vi "Teleop.vi"(10 "Match Info":T2={"Autonomous Elapsed Seconds"=0.0, "TeleOp Elapsed Seconds"=0.0, "Disabled Elapsed Seconds"=0.0, "Visited Autonomous"=FALSE, "Visited TeleOp"=FALSE, "Visited Disabled"=FALSE, "Autonomous Settings"={"Autonomous Style"=enum."Independent", "VI Refnum"=refnum}}, 11 "Call Context":T3) -> ()   [LabVIEW 2018]
doc: "This VI is called for each TeleOp packet received from the DS where the robot is not disabled. It is often used to read from the joysticks and update I/O or to update setpoints for timed control loops. It should complete and return within 20 milliseconds or it may miss DS packets."
uses:
  <vilib>/Rock Robotics/WPI/DriverStation/WPI_DriverStationDerivedRobotMode.ctl
  <vilib>/Rock Robotics/WPI/DriverStation/WPI_DriverStationMatch Info.ctl
  <vilib>/Rock Robotics/WPI/ThirdParty/Phoenix-LabVIEW/Motor Controller/Controls/CTRE_Phoenix_MotorControl_ControlMode.ctl
  <vilib>/Rock Robotics/WPI/Solenoid/WPI_SolenoidValue.ctl
  <vilib>/Rock Robotics/WPI/Utilities/WPI_GetSetVariantRefNum.vi
  <vilib>/Rock Robotics/WPI/ThirdParty/Phoenix-LabVIEW/Motor Controller/Get/CTRE_Phoenix_MotorController_GetSelectedSensorData.vi
  <vilib>/Rock Robotics/WPI/Solenoid/WPI_SolenoidSetEnum.vi
  <vilib>/Rock Robotics/Network Tables/NT Read Number.vi
panel:
  in  "FollowerLeft":dbl(slide) scale=-1.0..1.0
  in  "spark6":dbl(slide) scale=-1.0..1.0
  in  "Send LED Byte":bool
  in  "LED Byte":string
  out "Num Bytes Written":u32
  out "Operator Axis 4":dbl(slide) scale=-1.0..1.0
  out "Operator Buttons":bool[](array[boolean])
  out "Operator Axis 3":dbl(slide) scale=-1.0..1.0
  out "Operator Axis 2":dbl(slide) scale=-1.0..1.0
  out "Operator Axis 1":dbl(slide) scale=-1.0..1.0
  out "Image Out":T1(plugin-control)
  out "spark6encoder":dbl
  out "spark5encoder":dbl
  out "MasterLeft":dbl
  out "FollowerLeft":dbl
  out "MasterRight":dbl
  out "FollowerRight":dbl
  out "Keyboard Data":dbl
  out "HorseRight":i32
  out "ElevatorLeft":i32
  out "IntakeWrist":i32
  in  "Butterfly Drive Control":bool
  in  "Individual\nControl":bool
  in  "Test Run":bool
  in  "CargoKicker":bool
  in  "HorseDriveHatch":bool
  in  "Hatch":bool
  in  "Butterfly":bool
  in  "HorseLift":dbl(slide) scale=-1.0..1.0
  in  "IntakeWheels":dbl(slide) scale=-1.0..1.0
  in  "IntakeWrist":dbl(slide) scale=-1.0..1.0
  in  "ElevatorRight":dbl(slide) scale=-1.0..1.0
  in  "ElevatorLeft":dbl(slide) scale=-1.0..1.0
  in  "OuterStageDrive":dbl(slide) scale=-1.0..1.0
  in  "spark5":dbl(slide) scale=-1.0..1.0
  in  "MasterLeft":dbl(slide) scale=-1.0..1.0
  in  "MasterRight":dbl(slide) scale=-1.0..1.0
  in  "FollowerRight":dbl(slide) scale=-1.0..1.0
  # "TO DO LIST:\nUpdate all Talons and Victors\nto most recent firmware version\n4.17 for both controllers, firmware\nis located under 2019 firmware folder.\n\nID all motor controllers. Current code\nassumes the following ID's:\n0/1=LeftDrive\n2/3=RightDrive\n4=ButterflyLeft\n5=ButterflyRight\n6=OuterStage\n7=ElevatorLeft\n8=ElevatorRight\n9=IntakeWrist\n10=IntakeWheelse\n11=HorseDriveLeft\n12=HorseDriveRight\n\nVerify solenoid and PCM ID's, current\ncode assumes the following ID's:\n15=PCM\nSolenoid 0/1=Butterfly (dbl)\nSolenoid 2/3=Shift (dbl)\nSolenoid 4=Hatch (sngle)\nSolenoid 5=HorseDriveHatch (sngle)\nSolenoid 6=CargoKicker (sngle)"
  # "ADDITIONAL INFORMATION:\nCurrent code assumes all Talons for \nnon-drive-train motors. If some are\nVictors you only need to replace the open\nTalon VI's in BEGIN, all other VI's, such as\nset value, get value, refnum set/get, etc. \nare the same between Victor's or Talons.\n\nCurrent code has inverted the following:\nspark1\nspark2\nspark5\nElevatorRight\nHorseDriveRight\n\nThe main robot code uses the same\nbegin and finish code as the test project,\nTele-op however looks very different \nand uses keyboard based operator\nstation, if ready switch the operator station\nto a standard joystick copying off of the \nexisting joystick code. In addition, in the \nteleop there are two disabled VI's, the lower\none moved the elevator to a set encoder \nvalue and the other is a line following\ntest program. Both are completly untested\nfirst drafts use with caution. They are the \nlowest priorty to test."
  # "Controls main drive REV motors. 0 means\nno motor power, -1 means full reverse,1 means full \nforward. Spark 0-1 should ber ight drive, Spark 2-3 \nshould be left drive, Spark 4-5 should be butterfly \ndrive, with 4 being the left one.If individual control \nis TRUE, each slider controls that motor. If individual \ncontrol is FALSE, the slider becomes an indicator that \ndisplays percent output each motor is getting from \nthe joystick."
  # "Boolean control for\neach solenoid:\nTRUE: solenoid runs forward\nif doubleacting, or on if single\nacting. Should extend the piston.\nFALSE: Solenoid runs reverse if \ndoubleacting, or off if single\nacting, should withdraw the piston."
  # "Displays all axis from the operator station"
  # "Displays operator\nstation button\nvalues."
  # "Displays image fed into teleop from vision processing.VI"
  # "All encoder data from each\nREV Motor internal encoder"
  # "Controls LED signals"
  # "Sliders control talon motors, 0 means\nno motor power, -1 means full reverse,\n1 means full forward. \nIf Individual control is TRUE, this controls\neach specific motor, ignoring the other\nCAUTION,\nthis can damage gearboxes by running motors\nagainst each other\nIf Individual motor if FALSE, left (such as ElevatorLeft)\nmotor controls instead follow the right input."
  # "Test Run:\nFALSE: all functionality is disabled.\nTRUE: Allows robot control\n\nIndividiual Control\nFALSE: Controls elevator and horse\ndrive as one entity using the right\ninput, also drives the robot using\njoystick information.\nTRUE: Controls each motor directly\nand independitly from the others, CAUTION,\nthis can damage gearboxes by running motors\nagainst each other.\n\nButterfly Drive Control (Only has effect if\nIndividual control is FALSE).\nTRUE: Joystick control powers butterfly drive\nFALSE: Joystick control powers standard drive."
  # "All mag encoder data recieved from the robot, alongside\ncurrent keyboard data detected from dashboard."
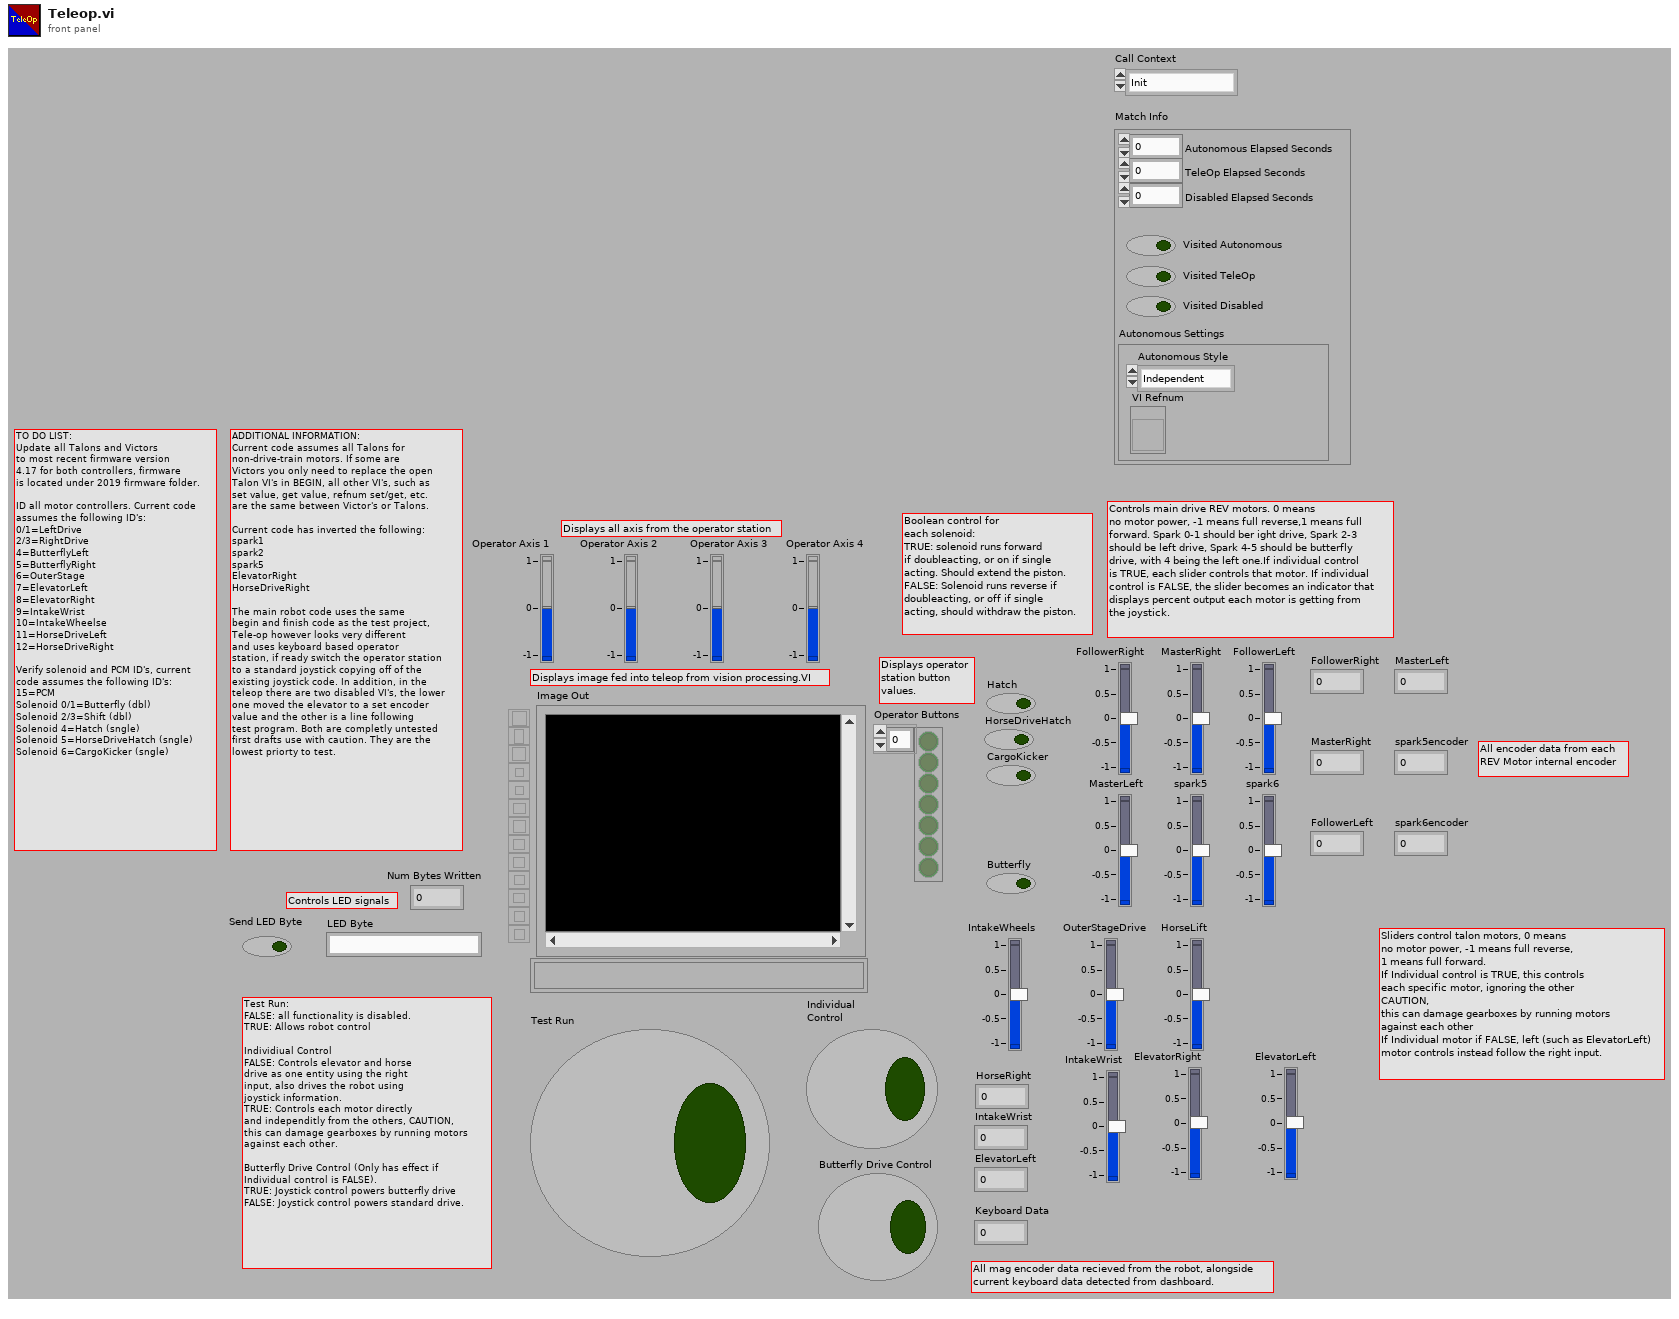
[diagram p1: front panel]
types:
  T1 = typedef "IMAQ Image.ctl" = refnum<image>
  T2 = typedef "WPI_DriverStationMatch Info.ctl" = cluster{"Autonomous Elapsed Seconds":dbl, "TeleOp Elapsed Seconds":dbl, "Disabled Elapsed Seconds":dbl, "Visited Autonomous":bool, "Visited TeleOp":bool, "Visited Disabled":bool, "Autonomous Settings":cluster{"Autonomous Style":enum16{"Iterative", "Independent"}, "VI Refnum":refnum<vi>}}
  T3 = typedef "WPI_DriverStationDerivedRobotMode.ctl" = enum16{"Init", "Execute", "Stop"}
  T4 = typedef "WPI_SerialPortRef.ctl" = cluster{"DevStatus":errorcluster, "Serial Port Name":refnum<visa-resource-name>}
  T5 = typedef "WPI_SolenoidValue.ctl" = enum16{"Off", "On", "Forward", "Reverse"}
  T6 = typedef "CTRE_Phoenix_MotorControl_ControlMode.ctl" = u16
  T7 = typedef "WPI_MotorControlDeviceRef.ctl" = cluster{"DeviceStatus":errorcluster, "Type":T8, "PWM":cluster{"PWM Channel":T9, "DeadBand":T10}, "CAN":cluster{"Device Number":u8, "SetOutput VI Ref":variant, "GetOutput VI Ref":variant, "Enable VI Ref":variant, "Disable VI Ref":variant, "Data":variant}, "Invert":bool, "DIO PWM":cluster{"PWM \"Enable\" Channel":T9, "DIOChannel":T11, "PWM Rate":dbl}}
  T8 = typedef "WPI_MotorControlType.ctl" = enum16{"PWM", "CAN", "DIO PWM"}
  T9 = typedef "FPGA_DIOPWMChannel.ctl" = enum8{"PWM 0", "PWM 1", "PWM 2", "PWM 3", "PWM 4", "PWM 5", "PWM 6", "PWM 7", "PWM 8", "PWM 9", "PWM MXP 0", "PWM MXP 1", "PWM MXP 2", "PWM MXP 3", "PWM MXP 4", "PWM MXP 5", "PWM MXP 6", "PWM MXP 7", "PWM MXP 8", "PWM MXP 9", "Invalid"}
  T10 = typedef "WPI_PWMDeadband.ctl" = cluster{"Name":string, "maxPositivePwm":i32, "minPositivePwm":i32, "centerPwm":i32, "maxNegativePwm":i32, "minNegativePwm":i32, "angularRange":u16}
  T11 = typedef "FPGA_DIOChannel.ctl" = enum8{"DIO 0", "DIO 1", "DIO 2", "DIO 3", "DIO 4", "DIO 5", "DIO 6", "DIO 7", "DIO 8", "DIO 9", "DIO MXP 0", "DIO MXP 1", "DIO MXP 2", "DIO MXP 3", "DIO MXP 4", "DIO MXP 5", "DIO MXP 6", "DIO MXP 7", "DIO MXP 8", "DIO MXP 9", "DIO MXP 10", "DIO MXP 11", "DIO MXP 12", "DIO MXP 13", "DIO MXP 14", "DIO MXP 15", "SPI Port CS1", "SPI Port CS2", "SPI Port CS3", "SPI Port MISO", "SPI Port MOSI", "Invalid"}
  T12 = typedef "WPI_JoystickDevRef.ctl" = cluster{"Device":T13}
  T13 = typedef "WPI_JoystickDeviceEnum.ctl" = enum16{"USB 0", "USB 1", "USB 2", "USB 3", "USB 4", "USB 5"}
  T14 = typedef "WPI_CameraDevRef.ctl" = cluster{"Camera Address":string, "CameraStatus":errorcluster}
  T15 = typedef "WPI_SolenoidDevRef.ctl" = cluster{"DevStatus":errorcluster, "Pneumatics Control Module":u8, "Forward Solenoid Channel":T16, "Reverse Solenoid Channel":T16}
  T16 = typedef "WPI_SolenoidChannel.ctl" = enum8{"Solenoid 0", "Solenoid 1", "Solenoid 2", "Solenoid 3", "Solenoid 4", "Solenoid 5", "Solenoid 6", "Solenoid 7", "Invalid"}
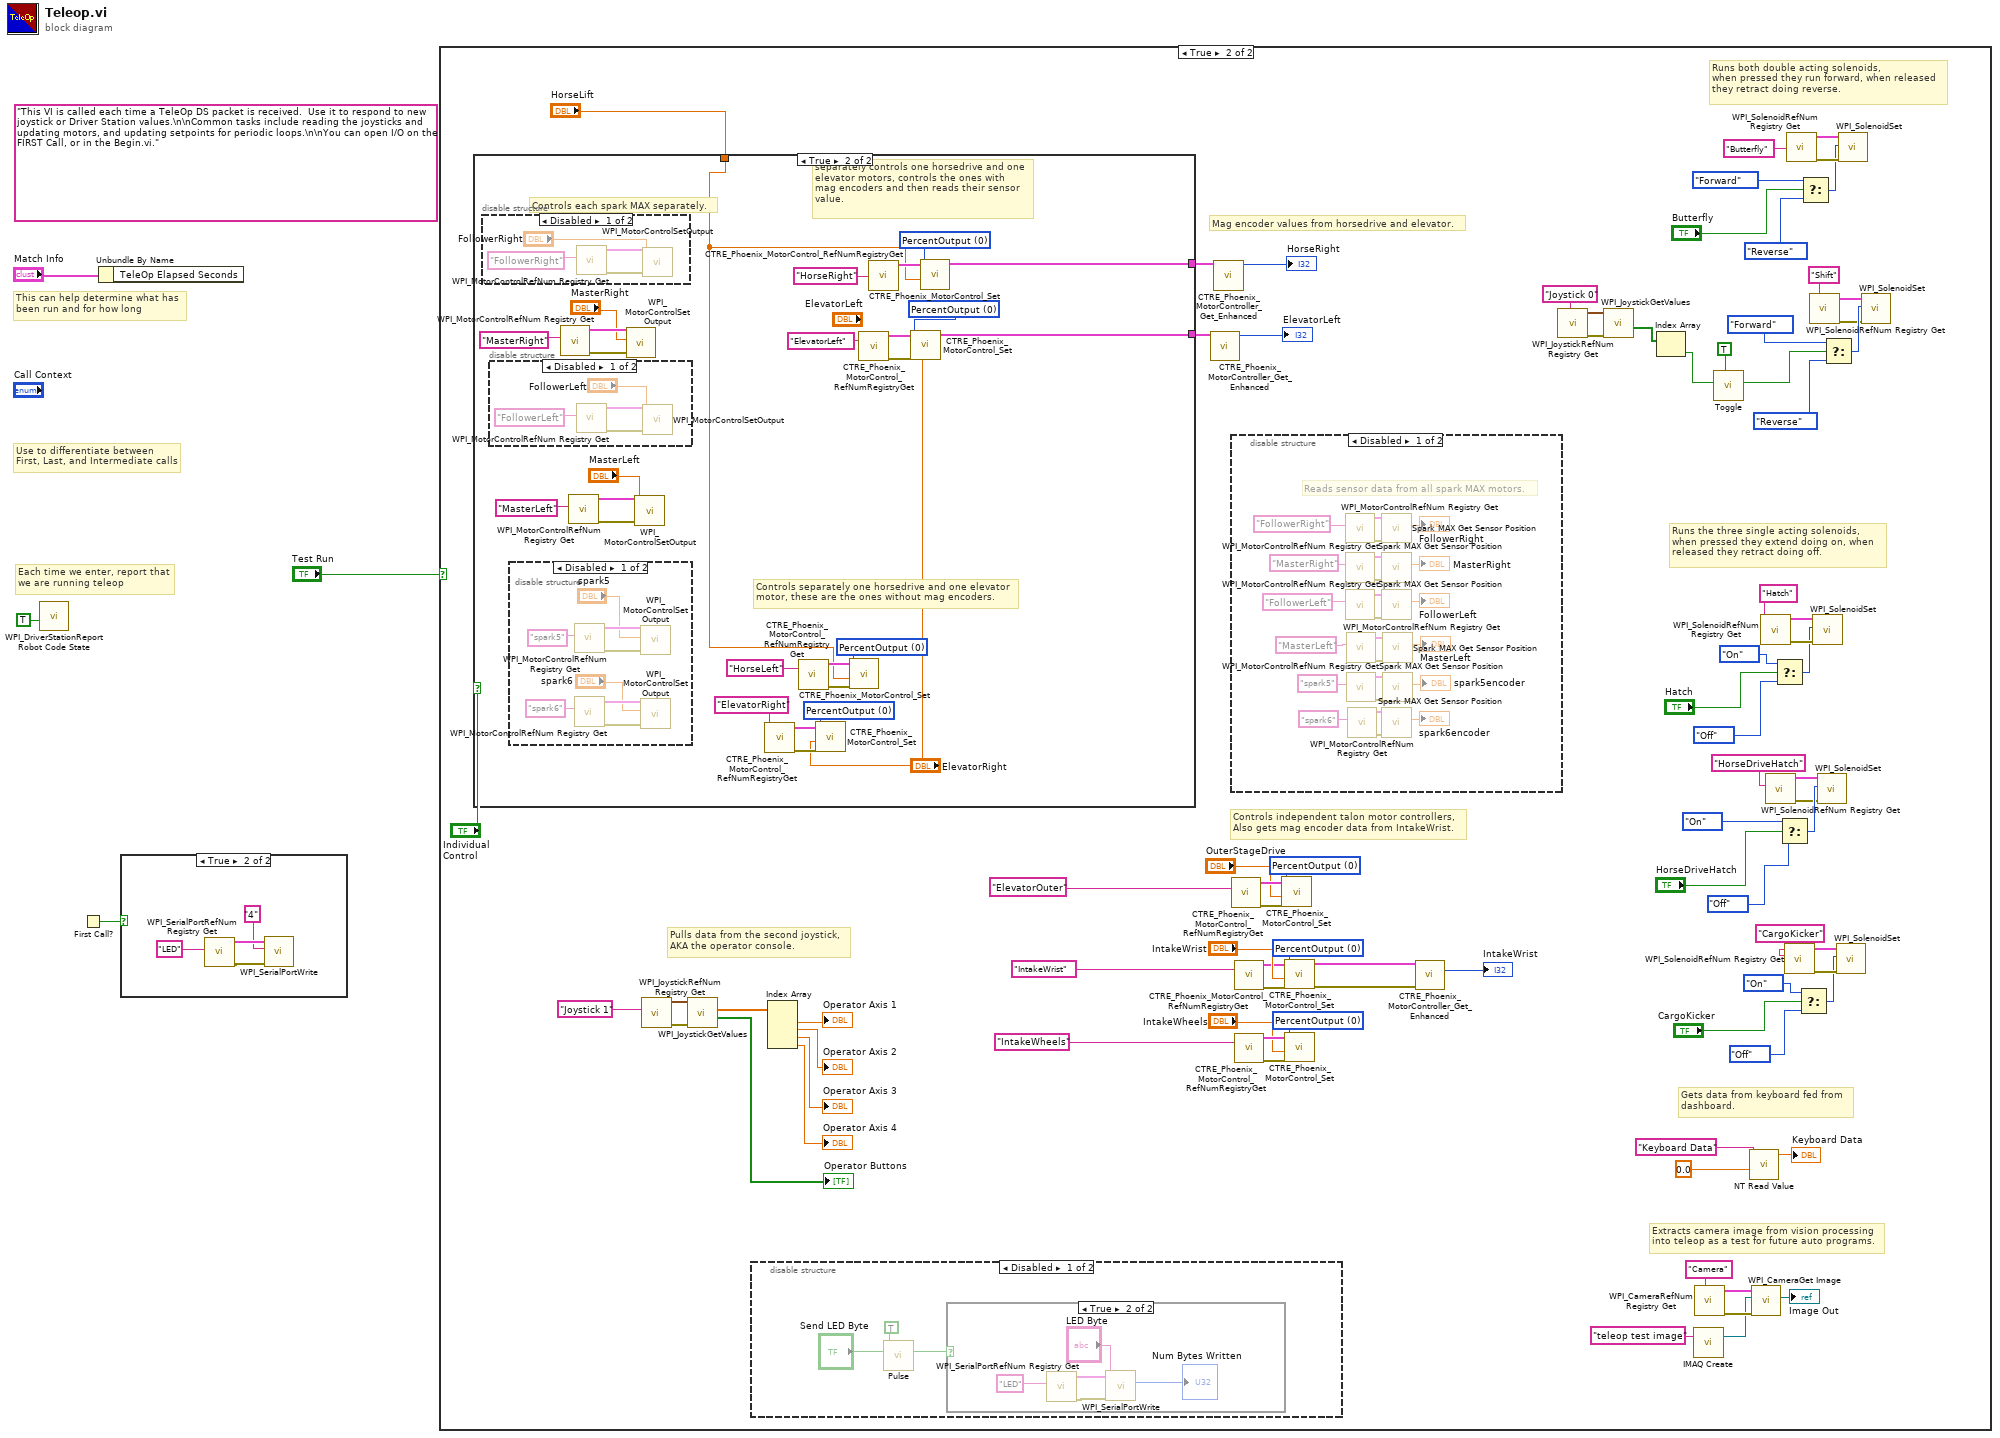
[diagram p0: block diagram]
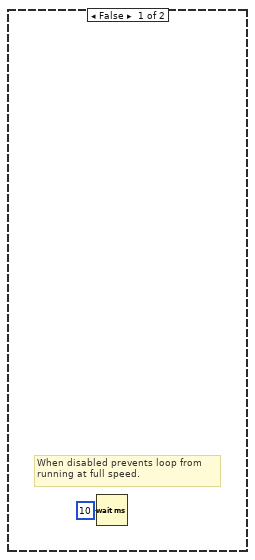
[diagram p3: hidden frame]
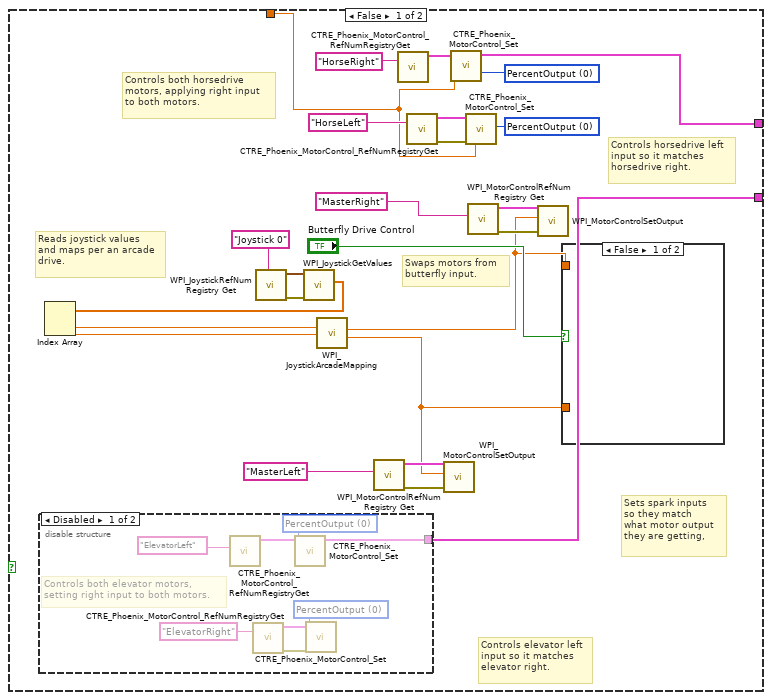
[diagram p7: hidden frame]
diagram:
  (unwired) "This VI is called each time a TeleOp DS packet is received.  Use it to respond to new joystick or Driver Station values.\n\nCommon tasks include reading the joysticks and updating motors, and updating setpoints for periodic loops.\n\nYou can open I/O on the FIRST Call, or in the Begin.vi."
  # "Each time we enter, report that\nwe are running teleop"
  # "Use to differentiate between\nFirst, Last, and Intermediate calls"
  # "This can help determine what has\nbeen run and for how long"
  n1 = call <vilib>:"WPI_DriverStationReport Robot Code State.vi"("TeleOp"=TRUE ("Autonomous")) -> ()  [unwired: 10 in, 1 out]
  n2 = First Call?() -> (First Call?: T/F=w1:bool)
  n3 = Unbundle By Name("Match Info") -> ()  [unwired: 1 out]
  n4 = case shown="True" w1 {
    frame False {
    }
    frame True {
      n5 = call <vilib>:"WPI_SerialPortRefNum Registry Get.vi"("refnum name"="LED") -> ("error out"=w5:errorcluster, "SerialPortRef"=w7:T4)  [unwired: 9 in]
      n6 = call <vilib>:"WPI_SerialPortWrite.vi"("error in (no error)"=w5, "Buffer"="4", "SerialPortRef"=w7) -> ()  [unwired: 6 in, 3 out]
    }
  }
  n7 = case shown="True" "Test Run" {
    frame False {
      # "When disabled prevents loop from\nrunning at full speed."
      n8 = Wait (ms)(milliseconds to wait=u32 10) -> ()  [unwired: 1 out]
    }
    frame True {
      w67 = T6 0 items=["PercentOutput"=0, "Position"=1, "Velocity"=2, "Current"=3, "Follower"=5, "MotionProfile"=6, "MotionMagic"=7, "MotionProfileArc"=10, "Disabled"=15] ("Control Mode")
      w72 = T6 0 items=["PercentOutput"=0, "Position"=1, "Velocity"=2, "Current"=3, "Follower"=5, "MotionProfile"=6, "MotionMagic"=7, "MotionProfileArc"=10, "Disabled"=15] ("Control Mode")
      w77 = T6 0 items=["PercentOutput"=0, "Position"=1, "Velocity"=2, "Current"=3, "Follower"=5, "MotionProfile"=6, "MotionMagic"=7, "MotionProfileArc"=10, "Disabled"=15] ("Control Mode")
      # "Mag encoder values from horsedrive and elevator."
      # "Extracts camera image from vision processing\ninto teleop as a test for future auto programs."
      # "Gets data from keyboard fed from\ndashboard."
      # "Runs both double acting solenoids,\nwhen pressed they run forward, when released\nthey retract doing reverse."
      # "Controls independent talon motor controllers,\nAlso gets mag encoder data from IntakeWrist."
      # "Pulls data from the second joystick,\nAKA the operator console."
      # "Runs the three single acting solenoids,\nwhen pressed they extend doing on, when\nreleased they retract doing off."
      n9 = case shown="True" "Individual\nControl" {
        tunnel: "HorseLift" -> [w127 w167]
        tunnel: [w131 w184] -> w90
        tunnel: [w132 w183] -> w89
        frame False {
          w134 = T6 0 items=["PercentOutput"=0, "Position"=1, "Velocity"=2, "Current"=3, "Follower"=5, "MotionProfile"=6, "MotionMagic"=7, "MotionProfileArc"=10, "Disabled"=15] ("Control Mode")
          w138 = T6 0 items=["PercentOutput"=0, "Position"=1, "Velocity"=2, "Current"=3, "Follower"=5, "MotionProfile"=6, "MotionMagic"=7, "MotionProfileArc"=10, "Disabled"=15] ("Control Mode")
          # "Sets spark inputs\nso they match\nwhat motor output\nthey are getting,"
          # "Controls horsedrive left\ninput so it matches \nhorsedrive right."
          # "Controls elevator left\ninput so it matches \nelevator right."
          # "Swaps motors from\nbutterfly input."
          # "Reads joystick values\nand maps per an arcade\ndrive."
          # "Controls both horsedrive\nmotors, applying right input\nto both motors."
          n10 = disable-structure shown="Disabled" {
            disable-tunnel: [w150 _] -> w131
            frame Disabled {
              w154 = T6 0 items=["PercentOutput"=0, "Position"=1, "Velocity"=2, "Current"=3, "Follower"=5, "MotionProfile"=6, "MotionMagic"=7, "MotionProfileArc"=10, "Disabled"=15] ("Control Mode")
              w157 = T6 0 items=["PercentOutput"=0, "Position"=1, "Velocity"=2, "Current"=3, "Follower"=5, "MotionProfile"=6, "MotionMagic"=7, "MotionProfileArc"=10, "Disabled"=15] ("Control Mode")
              # "Controls both elevator motors,\nsetting right input to both motors."
              n11 = call <vilib>:"CTRE_Phoenix_MotorControl_RefNumRegistryGet.vi"("refnum name"="ElevatorLeft") -> ("PhoenixMotorControlDevRef"=w151:T7)  [unwired: 9 in, 1 out]
              n12 = call <vilib>:"CTRE_Phoenix_MotorControl_RefNumRegistryGet.vi"("refnum name"="ElevatorRight") -> ("error out"=w156:errorcluster, "PhoenixMotorControlDevRef"=w155:T7)  [unwired: 9 in]
              n13 = call <vilib>:"CTRE_Phoenix_MotorControl_Set.vi"("Control Mode"=w157, "PhoenixMotorControlDevRef"=w151) -> ("PhoenixMotorControlDevRef"=w150:T7)  [unwired: 8 in, 1 out]
              n14 = call <vilib>:"CTRE_Phoenix_MotorControl_Set.vi"("error in (no error)"=w156, "Control Mode"=w154, "PhoenixMotorControlDevRef"=w155) -> ()  [unwired: 7 in, 2 out]
            }
            frame Enabled {
            }
          }
          n15 = call <vilib>:"WPI_JoystickRefNum Registry Get.vi"("refnum name"="Joystick 0") -> ("error out"=w145:errorcluster, "JoystickDevRef"=w144:T12)  [unwired: 9 in]
          n16 = call <vilib>:"WPI_JoystickGetValues.vi"("error in (no error)"=w145, "JoystickDevRef"=w144) -> ("Axes"=w142:dbl[])  [unwired: 5 in, 4 out]
          n17 = Index Array(array=w142) -> (element #1=w141:dbl, element #2=w140:dbl)  [unwired: 2 in]
          n18 = call <vilib>:"WPI_JoystickArcadeMapping.vi"("Y axis value"=w140, "X axis value"=w141) -> ("Right Motor Value"=w128:dbl, "Left Motor Value"=w129:dbl)  [unwired: 8 in]
          n19 = call <vilib>:"WPI_MotorControlRefNum Registry Get.vi"("refnum name"="MasterLeft") -> ("error out"=w149:errorcluster, "MotorControlDevRef"=w148:T7)  [unwired: 9 in]
          n20 = call <vilib>:"CTRE_Phoenix_MotorControl_RefNumRegistryGet.vi"("refnum name"="HorseRight") -> ("PhoenixMotorControlDevRef"=w135:T7)  [unwired: 9 in, 1 out]
          n21 = call <vilib>:"CTRE_Phoenix_MotorControl_RefNumRegistryGet.vi"("refnum name"="HorseLeft") -> ("error out"=w136:errorcluster, "PhoenixMotorControlDevRef"=w137:T7)  [unwired: 9 in]
          n22 = call <vilib>:"WPI_MotorControlSetOutput.vi"("error in (no error)"=w149, "Output"=w128, "MotorControlDevRef"=w148) -> ()  [unwired: 6 in, 3 out]
          n23 = call <vilib>:"CTRE_Phoenix_MotorControl_Set.vi"("Output"=w127, "Control Mode"=w134, "PhoenixMotorControlDevRef"=w135) -> ("PhoenixMotorControlDevRef"=w132:T7)  [unwired: 7 in, 1 out]
          n24 = call <vilib>:"CTRE_Phoenix_MotorControl_Set.vi"("error in (no error)"=w136, "Output"=w127, "Control Mode"=w138, "PhoenixMotorControlDevRef"=w137) -> ()  [unwired: 6 in, 2 out]
          n25 = call <vilib>:"WPI_MotorControlRefNum Registry Get.vi"("refnum name"="MasterRight") -> ("error out"=w146:errorcluster, "MotorControlDevRef"=w147:T7)  [unwired: 9 in]
          n26 = call <vilib>:"WPI_MotorControlSetOutput.vi"("error in (no error)"=w146, "Output"=w129, "MotorControlDevRef"=w147) -> ()  [unwired: 6 in, 3 out]
          n27 = case shown="False" "Butterfly Drive Control" {
            tunnel: w129 -> [_ _]
            tunnel: w128 -> [_ _]
            frame False {
            }
            frame True {
            }
          }
        }
        frame True {
          w161 = T6 0 items=["PercentOutput"=0, "Position"=1, "Velocity"=2, "Current"=3, "Follower"=5, "MotionProfile"=6, "MotionMagic"=7, "MotionProfileArc"=10, "Disabled"=15] ("Control Mode")
          w164 = T6 0 items=["PercentOutput"=0, "Position"=1, "Velocity"=2, "Current"=3, "Follower"=5, "MotionProfile"=6, "MotionMagic"=7, "MotionProfileArc"=10, "Disabled"=15] ("Control Mode")
          w178 = T6 0 items=["PercentOutput"=0, "Position"=1, "Velocity"=2, "Current"=3, "Follower"=5, "MotionProfile"=6, "MotionMagic"=7, "MotionProfileArc"=10, "Disabled"=15] ("Control Mode")
          w181 = T6 0 items=["PercentOutput"=0, "Position"=1, "Velocity"=2, "Current"=3, "Follower"=5, "MotionProfile"=6, "MotionMagic"=7, "MotionProfileArc"=10, "Disabled"=15] ("Control Mode")
          # "Controls separately one horsedrive and one elevator\nmotor, these are the ones without mag encoders."
          # "separately controls one horsedrive and one\nelevator motors, controls the ones with\nmag encoders and then reads their sensor\nvalue."
          # "Controls each spark MAX separately."
          n28 = disable-structure shown="Disabled" {
            frame Disabled {
              n29 = call <vilib>:"WPI_MotorControlRefNum Registry Get.vi"("refnum name"="FollowerRight") -> ("error out"=w187:errorcluster, "MotorControlDevRef"=w186:T7)  [unwired: 9 in]
              n30 = call <vilib>:"WPI_MotorControlSetOutput.vi"("error in (no error)"=w187, "Output"="FollowerRight", "MotorControlDevRef"=w186) -> ()  [unwired: 6 in, 3 out]
            }
            frame Enabled {
            }
          }
          n31 = disable-structure shown="Disabled" {
            frame Disabled {
              n32 = call <vilib>:"WPI_MotorControlRefNum Registry Get.vi"("refnum name"="FollowerLeft") -> ("error out"=w191:errorcluster, "MotorControlDevRef"=w190:T7)  [unwired: 9 in]
              n33 = call <vilib>:"WPI_MotorControlSetOutput.vi"("error in (no error)"=w191, "Output"="FollowerLeft", "MotorControlDevRef"=w190) -> ()  [unwired: 6 in, 3 out]
            }
            frame Enabled {
            }
          }
          n34 = disable-structure shown="Disabled" {
            frame Disabled {
              n35 = call <vilib>:"WPI_MotorControlRefNum Registry Get.vi"("refnum name"="spark5") -> ("error out"=w199:errorcluster, "MotorControlDevRef"=w200:T7)  [unwired: 9 in]
              n36 = call <vilib>:"WPI_MotorControlRefNum Registry Get.vi"("refnum name"="spark6") -> ("error out"=w196:errorcluster, "MotorControlDevRef"=w195:T7)  [unwired: 9 in]
              n37 = call <vilib>:"WPI_MotorControlSetOutput.vi"("error in (no error)"=w199, "Output"="spark5", "MotorControlDevRef"=w200) -> ()  [unwired: 6 in, 3 out]
              n38 = call <vilib>:"WPI_MotorControlSetOutput.vi"("error in (no error)"=w196, "Output"="spark6", "MotorControlDevRef"=w195) -> ()  [unwired: 6 in, 3 out]
            }
            frame Enabled {
            }
          }
          n39 = call <vilib>:"WPI_MotorControlRefNum Registry Get.vi"("refnum name"="MasterRight") -> ("error out"=w174:errorcluster, "MotorControlDevRef"=w173:T7)  [unwired: 9 in]
          n40 = call <vilib>:"WPI_MotorControlRefNum Registry Get.vi"("refnum name"="MasterLeft") -> ("error out"=w171:errorcluster, "MotorControlDevRef"=w170:T7)  [unwired: 9 in]
          n41 = call <vilib>:"WPI_MotorControlSetOutput.vi"("error in (no error)"=w174, "Output"="MasterRight", "MotorControlDevRef"=w173) -> ()  [unwired: 6 in, 3 out]
          n42 = call <vilib>:"WPI_MotorControlSetOutput.vi"("error in (no error)"=w171, "Output"="MasterLeft", "MotorControlDevRef"=w170) -> ()  [unwired: 6 in, 3 out]
          n43 = call <vilib>:"CTRE_Phoenix_MotorControl_RefNumRegistryGet.vi"("refnum name"="ElevatorRight") -> ("error out"=w166:errorcluster, "PhoenixMotorControlDevRef"=w165:T7)  [unwired: 9 in]
          n44 = call <vilib>:"CTRE_Phoenix_MotorControl_RefNumRegistryGet.vi"("refnum name"="HorseLeft") -> ("error out"=w176:errorcluster, "PhoenixMotorControlDevRef"=w177:T7)  [unwired: 9 in]
          n45 = call <vilib>:"CTRE_Phoenix_MotorControl_Set.vi"("error in (no error)"=w166, "Output"="ElevatorRight", "Control Mode"=w164, "PhoenixMotorControlDevRef"=w165) -> ()  [unwired: 6 in, 2 out]
          n46 = call <vilib>:"CTRE_Phoenix_MotorControl_Set.vi"("error in (no error)"=w176, "Output"=w167, "Control Mode"=w178, "PhoenixMotorControlDevRef"=w177) -> ()  [unwired: 6 in, 2 out]
          n47 = call <vilib>:"CTRE_Phoenix_MotorControl_RefNumRegistryGet.vi"("refnum name"="ElevatorLeft") -> ("error out"=w159:errorcluster, "PhoenixMotorControlDevRef"=w160:T7)  [unwired: 9 in]
          n48 = call <vilib>:"CTRE_Phoenix_MotorControl_RefNumRegistryGet.vi"("refnum name"="HorseRight") -> ("PhoenixMotorControlDevRef"=w182:T7)  [unwired: 9 in, 1 out]
          n49 = call <vilib>:"CTRE_Phoenix_MotorControl_Set.vi"("error in (no error)"=w159, "Output"="ElevatorRight", "Control Mode"=w161, "PhoenixMotorControlDevRef"=w160) -> ("PhoenixMotorControlDevRef"=w184:T7)  [unwired: 6 in, 1 out]
          n50 = call <vilib>:"CTRE_Phoenix_MotorControl_Set.vi"("Output"=w167, "Control Mode"=w181, "PhoenixMotorControlDevRef"=w182) -> ("PhoenixMotorControlDevRef"=w183:T7)  [unwired: 7 in, 1 out]
        }
      }
      n51 = call <vilib>:"WPI_JoystickRefNum Registry Get.vi"("refnum name"="Joystick 1") -> ("error out"=w86:errorcluster, "JoystickDevRef"=w88:T12)  [unwired: 9 in]
      n52 = call <vilib>:"WPI_JoystickGetValues.vi"("error in (no error)"=w86, "JoystickDevRef"=w88) -> ("Buttons"=→"Operator Buttons":bool[], "Axes"=w85:dbl[])  [unwired: 5 in, 3 out]
      n53 = disable-structure shown="Disabled" {
        frame Disabled {
          n54 = call "Pulse.vi"("Input"="Send LED Byte", "Rising Edge?"=TRUE) -> ("Output"=w119:bool)  [unwired: 9 in]
          n55 = case shown="True" w119 {
            frame False {
            }
            frame True {
              n56 = call <vilib>:"WPI_SerialPortRefNum Registry Get.vi"("refnum name"="LED") -> ("error out"=w122:errorcluster, "SerialPortRef"=w123:T4)  [unwired: 9 in]
              n57 = call <vilib>:"WPI_SerialPortWrite.vi"("error in (no error)"=w122, "Buffer"="LED Byte", "SerialPortRef"=w123) -> ("Num Bytes Written"=→"Num Bytes Written":u32)  [unwired: 6 in, 2 out]
            }
          }
        }
        frame Enabled {
        }
      }
      n58 = Index Array(array=w85) -> (element #1=→"Operator Axis 1":dbl, element #2=→"Operator Axis 2":dbl, element #3=→"Operator Axis 3":dbl, element #4=→"Operator Axis 4":dbl)  [unwired: 4 in]
      n59 = call-poly <vilib>:"CTRE_Phoenix_MotorController_Get_Enhanced.vi"("PhoenixMotorControlDevRef"=w90) -> ("Position (Raw Sensor Units)"=→"ElevatorLeft":i32)  [unwired: 11 in, 3 out]
      n60 = call-poly <vilib>:"CTRE_Phoenix_MotorController_Get_Enhanced.vi"("PhoenixMotorControlDevRef"=w89) -> ("Position (Raw Sensor Units)"=→"HorseRight":i32)  [unwired: 11 in, 3 out]
      n61 = disable-structure shown="Disabled" {
        frame Disabled {
          # "Reads sensor data from all spark MAX motors."
          n62 = call <vilib>:"WPI_MotorControlRefNum Registry Get.vi"("refnum name"="FollowerRight") -> ("error out"=w98:errorcluster, "MotorControlDevRef"=w104:T7)  [unwired: 9 in]
          n63 = call <vilib>:"WPI_MotorControlRefNum Registry Get.vi"("refnum name"="MasterRight") -> ("error out"=w97:errorcluster, "MotorControlDevRef"=w103:T7)  [unwired: 9 in]
          n64 = call <vilib>:"WPI_MotorControlRefNum Registry Get.vi"("refnum name"="FollowerLeft") -> ("error out"=w96:errorcluster, "MotorControlDevRef"=w102:T7)  [unwired: 9 in]
          n65 = call <vilib>:"WPI_MotorControlRefNum Registry Get.vi"("refnum name"="MasterLeft") -> ("error out"=w95:errorcluster, "MotorControlDevRef"=w101:T7)  [unwired: 9 in]
          n66 = call <vilib>:"WPI_MotorControlRefNum Registry Get.vi"("refnum name"="spark5") -> ("error out"=w94:errorcluster, "MotorControlDevRef"=w100:T7)  [unwired: 9 in]
          n67 = call <vilib>:"WPI_MotorControlRefNum Registry Get.vi"("refnum name"="spark6") -> ("error out"=w93:errorcluster, "MotorControlDevRef"=w99:T7)  [unwired: 9 in]
          n68 = call <vilib>:"Spark MAX Get Sensor Position.vi"("error in (no error)"=w98, "MotorControlDevRef in"=w104) -> ("Sensor Position"=→"FollowerRight":dbl)  [unwired: 6 in, 3 out]
          n69 = call <vilib>:"Spark MAX Get Sensor Position.vi"("error in (no error)"=w97, "MotorControlDevRef in"=w103) -> ("Sensor Position"=→"MasterRight":dbl)  [unwired: 6 in, 3 out]
          n70 = call <vilib>:"Spark MAX Get Sensor Position.vi"("error in (no error)"=w96, "MotorControlDevRef in"=w102) -> ("Sensor Position"=→"FollowerLeft":dbl)  [unwired: 6 in, 3 out]
          n71 = call <vilib>:"Spark MAX Get Sensor Position.vi"("error in (no error)"=w93, "MotorControlDevRef in"=w99) -> ("Sensor Position"=→"spark6encoder":dbl)  [unwired: 6 in, 3 out]
          n72 = call <vilib>:"Spark MAX Get Sensor Position.vi"("error in (no error)"=w95, "MotorControlDevRef in"=w101) -> ("Sensor Position"=→"MasterLeft":dbl)  [unwired: 6 in, 3 out]
          n73 = call <vilib>:"Spark MAX Get Sensor Position.vi"("error in (no error)"=w94, "MotorControlDevRef in"=w100) -> ("Sensor Position"=→"spark5encoder":dbl)  [unwired: 6 in, 3 out]
        }
        frame Enabled {
        }
      }
      n74 = call <vilib>:"CTRE_Phoenix_MotorControl_RefNumRegistryGet.vi"("refnum name"="ElevatorOuter") -> ("error out"=w79:errorcluster, "PhoenixMotorControlDevRef"=w78:T7)  [unwired: 9 in]
      n75 = call <vilib>:"CTRE_Phoenix_MotorControl_RefNumRegistryGet.vi"("refnum name"="IntakeWrist") -> ("error out"=w70:errorcluster, "PhoenixMotorControlDevRef"=w71:T7)  [unwired: 9 in]
      n76 = call <vilib>:"CTRE_Phoenix_MotorControl_RefNumRegistryGet.vi"("refnum name"="IntakeWheels") -> ("error out"=w69:errorcluster, "PhoenixMotorControlDevRef"=w68:T7)  [unwired: 9 in]
      n77 = call <vilib>:"CTRE_Phoenix_MotorControl_Set.vi"("error in (no error)"=w79, "Output"="OuterStageDrive", "Control Mode"=w77, "PhoenixMotorControlDevRef"=w78) -> ()  [unwired: 6 in, 2 out]
      n78 = call <vilib>:"CTRE_Phoenix_MotorControl_Set.vi"("error in (no error)"=w70, "Output"="IntakeWrist", "Control Mode"=w72, "PhoenixMotorControlDevRef"=w71) -> ("error out"=w63:errorcluster, "PhoenixMotorControlDevRef"=w64:T7)  [unwired: 6 in]
      n79 = call <vilib>:"CTRE_Phoenix_MotorControl_Set.vi"("error in (no error)"=w69, "Output"="IntakeWheels", "Control Mode"=w67, "PhoenixMotorControlDevRef"=w68) -> ()  [unwired: 6 in, 2 out]
      n80 = call-poly <vilib>:"CTRE_Phoenix_MotorController_Get_Enhanced.vi"("PhoenixMotorControlDevRef"=w64, "error in"=w63) -> ("Position (Raw Sensor Units)"=→"IntakeWrist":i32)  [unwired: 10 in, 3 out]
      n81 = call <vilib>:"WPI_JoystickRefNum Registry Get.vi"("refnum name"="Joystick 0") -> ("error out"=w18:errorcluster, "JoystickDevRef"=w19:T12)  [unwired: 9 in]
      n82 = call <vilib>:"WPI_JoystickGetValues.vi"("error in (no error)"=w18, "JoystickDevRef"=w19) -> ("Buttons"=w16:bool[])  [unwired: 5 in, 4 out]
      n83 = Index Array(array=w16) -> (element=w15:bool)  [unwired: 1 in]
      n84 = call "IMAQ Create"("Image Name"="teleop test image") -> ("New Image"=w21:T1)  [unwired: 4 in, 1 out]
      n85 = call <vilib>:"WPI_CameraRefNum Registry Get.vi"("refnum name"="Camera") -> ("error out"=w25:errorcluster, "CameraDevRef"=w24:T14)  [unwired: 9 in]
      n86 = call "Toggle.vi"("Control"=TRUE, "Input"=w15) -> ("Output"=w14:bool)  [unwired: 9 in]
      n87 = call-poly <vilib>:"NT Read Value.vi"("Default Value"=0.0, "Name"="Keyboard Data") -> ("Numeric"=→"Keyboard Data":dbl)  [unwired: 8 in, 1 out]
      n88 = call <vilib>:"WPI_CameraGet Image.vi"("error in (no error)"=w25, "Image"=w21, "CameraDevRef"=w24) -> ("Image Out"=→"Image Out":T1)  [unwired: 6 in, 2 out]
      n89 = call <vilib>:"WPI_SolenoidRefNum Registry Get.vi"("refnum name"="Hatch") -> ("error out"=w49:errorcluster, "SolenoidDevRef"=w48:T15)  [unwired: 9 in]
      n90 = call <vilib>:"WPI_SolenoidRefNum Registry Get.vi"("refnum name"="HorseDriveHatch") -> ("error out"=w37:errorcluster, "SolenoidDevRef"=w38:T15)  [unwired: 9 in]
      n91 = Select(t=WPI_SolenoidValue."On" ("Value"), s="Hatch", f=WPI_SolenoidValue."Off") -> (s? t:f=w43:T5)
      n92 = Select(t=WPI_SolenoidValue."On" ("Value"), s="HorseDriveHatch", f=WPI_SolenoidValue."Off") -> (s? t:f=w42:T5)
      n93 = call <vilib>:"WPI_SolenoidRefNum Registry Get.vi"("refnum name"="CargoKicker") -> ("error out"=w36:errorcluster, "SolenoidDevRef"=w35:T15)  [unwired: 9 in]
      n94 = call <vilib>:"WPI_SolenoidRefNum Registry Get.vi"("refnum name"="Butterfly") -> ("error out"=w62:errorcluster, "SolenoidDevRef"=w61:T15)  [unwired: 9 in]
      n95 = Select(t=WPI_SolenoidValue."On" ("Value"), s="CargoKicker", f=WPI_SolenoidValue."Off") -> (s? t:f=w31:T5)
      n96 = Select(t=WPI_SolenoidValue."Forward" ("Value"), s="Butterfly", f=WPI_SolenoidValue."Reverse") -> (s? t:f=w56:T5)
      n97 = call <vilib>:"WPI_SolenoidRefNum Registry Get.vi"("refnum name"="Shift") -> ("error out"=w50:errorcluster, "SolenoidDevRef"=w51:T15)  [unwired: 9 in]
      n98 = call-poly <vilib>:"WPI_SolenoidSet.vi"("error in (no error)"=w49, "Value"=w43, "SolenoidDevRef"=w48) -> ()  [unwired: 7 in, 2 out]
      n99 = call-poly <vilib>:"WPI_SolenoidSet.vi"("error in (no error)"=w37, "Value"=w42, "SolenoidDevRef"=w38) -> ()  [unwired: 7 in, 2 out]
      n100 = Select(t=WPI_SolenoidValue."Forward" ("Value"), s=w14, f=WPI_SolenoidValue."Reverse") -> (s? t:f=w55:T5)
      n101 = call-poly <vilib>:"WPI_SolenoidSet.vi"("error in (no error)"=w36, "Value"=w31, "SolenoidDevRef"=w35) -> ()  [unwired: 7 in, 2 out]
      n102 = call-poly <vilib>:"WPI_SolenoidSet.vi"("error in (no error)"=w62, "Value"=w56, "SolenoidDevRef"=w61) -> ()  [unwired: 7 in, 2 out]
      n103 = call-poly <vilib>:"WPI_SolenoidSet.vi"("error in (no error)"=w50, "Value"=w55, "SolenoidDevRef"=w51) -> ()  [unwired: 7 in, 2 out]
    }
  }
